vi "SaveConfigFile.vi"(8 "error in":errorcluster, 9 "ConnectConfig":T1={"IP Address"="", "Port"=102, "Timeout"=5000}, 10 "Model Name":string, 11 "Configuration":T2) -> (0 "error out":errorcluster)   [LabVIEW 2025, in "PLC_Module.lvlib" / "PLC_Module.lvclass"]
uses:
  PLC_Module.lvclass
  PLC_Data_Config.ctl
  PLC_Data.ctl
  PLC_Data_Type.ctl
  PLC_Connect_Config.ctl
  PLC_Config.ctl
  8819672f-02f5-46b1-a926-4b7b34d67a49.vi
  <vilib>/JDP Science/JSONtext/Variant to JSON Text.vi
  <vilib>/JDP Science/JSONtext/LVClass Serializer/JSONtext LVClass Serializer.lvclass
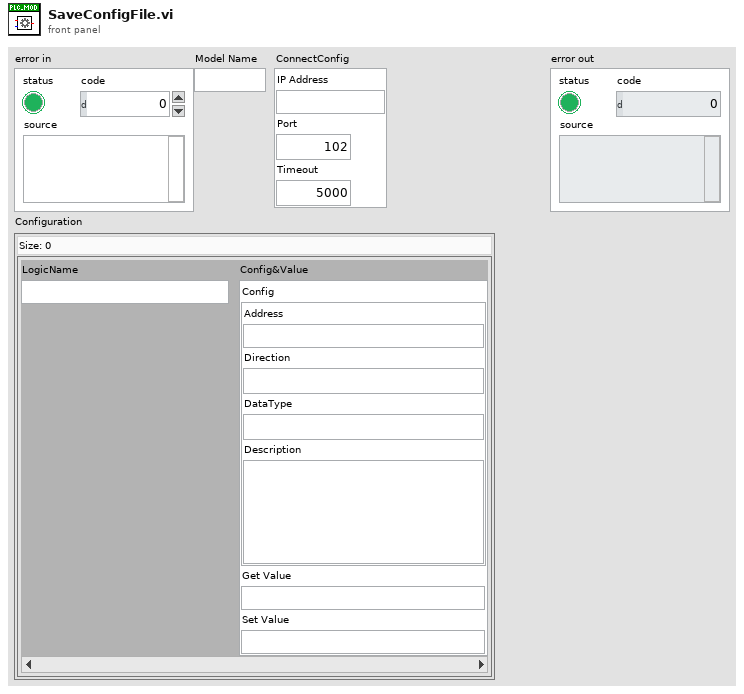
[diagram p1: front panel]
types:
  T1 = typedef "PLC_Module.lvlib/PLC_Module.lvclass/PLC_Connect_Config.ctl" = cluster{"IP Address":string, "Port":u16, "Timeout":i32}
  T2 = typedef "PLC_Module.lvlib/PLC_Module.lvclass/PLC_Data_Config.ctl" = map{string, cluster{"Config":T3, "Get Value":string, "Set Value":string}}
  T3 = typedef "PLC_Module.lvlib/PLC_Module.lvclass/PLC_Data.ctl" = cluster{"Address":string, "Direction":enum16{"PC->PLC", "PLC->PC"}, "DataType":T4, "Description":string}
  T4 = typedef "PLC_Module.lvlib/PLC_Module.lvclass/PLC_Data_Type.ctl" = enum16{"Boolean", "Single Float", "U8", "U32", "U32_Array", "String"}
  T5 = typedef "PLC_Module.lvlib/PLC_Module.lvclass/PLC_Config.ctl" = cluster{"ConnectConfig":T1, "DataConfiguration":T2}
  T6 = enum16{"open", "replace", "create", "open or create", "replace or create", "replace or create with confirmation"}
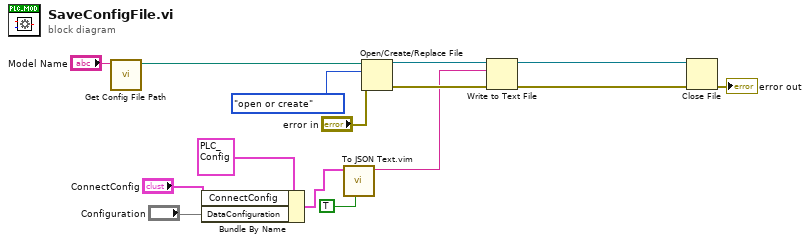
[diagram p0: block diagram]
diagram:
  n1 = call "Get Config File Path.vi"("Model Name"="Model Name") -> ("appended path"=w15:path)  [unwired: 10 in]
  n2 = Bundle By Name(cluster=T5 {"ConnectConfig"={"IP Address"="", "Port"=102, "Timeout"=5000}, "DataConfiguration"={}} ("PLC_Config"), "ConnectConfig"="ConnectConfig", "DataConfiguration"="Configuration") -> (w1:T5)
  n3 = call "To JSON Text.vim"("Pretty Print?"=TRUE, "Anything"=w1) -> ("<JSON>"=w7:string)  [unwired: 8 in, 1 out]
  n4 = Open/Create/Replace File(file path (use dialog)=w15, error in="error in", operation (0:open)=T6."open or create") -> (refnum out=w13:refnum<file>, error out=w12:errorcluster)  [unwired: 3 in, 1 out]
  n5 = Write to Text File(file (use dialog)=w13, text=w7, error in=w12) -> (refnum out=w11:refnum<file>, error out=w10:errorcluster)  [unwired: 1 in, 1 out]
  n6 = Close File(refnum=w11, error in=w10) -> (error out=→"error out":errorcluster)  [unwired: 1 out]
